vi "Generate Case Description.vi"(8 "error in (no error)":errorcluster, 10 "Test Case Result Out in":T1, 11 "Test Tree In":refnum<class "Test Result Tree.lvclass">) -> (0 "error out":errorcluster, 2 "Test Case Result Out out":T1, 3 "Test Tree Out":refnum<class "Test Result Tree.lvclass">)   [LabVIEW 2020, in "Test Result Tree.lvclass"]
uses:
  Framework/Helper Classes/Test Result Tree/Test Result Tree.lvclass
  Framework/Result Types/Case Result/Test Case Result.ctl
  Framework/Result Types/Method Result/Method Result.ctl
  Result/Status.ctl
  Framework/Result Types/Assertion Result/Assertion Result.ctl
  Framework/Result Types/Assertion Result/Public/TypeDefs/Assertion Type.ctl
  C:/Git/astemes-lunit/source/Framework/Helper Classes/Test Tree/Test Tree.lvclass
  Test Tree.lvclass/Test Tree.ctl
  Framework/Result Types/Case Result/Private/Count by Status.vi
  Framework/Result Types/Case Result/Test Case Result.lvlib
  Test Tree.lvclass
  Framework/Result Types/Assertion Result/Assertion Result.lvlib
  Framework/Result Types/Method Result/Method Result.lvlib
  Result/Result.lvlib
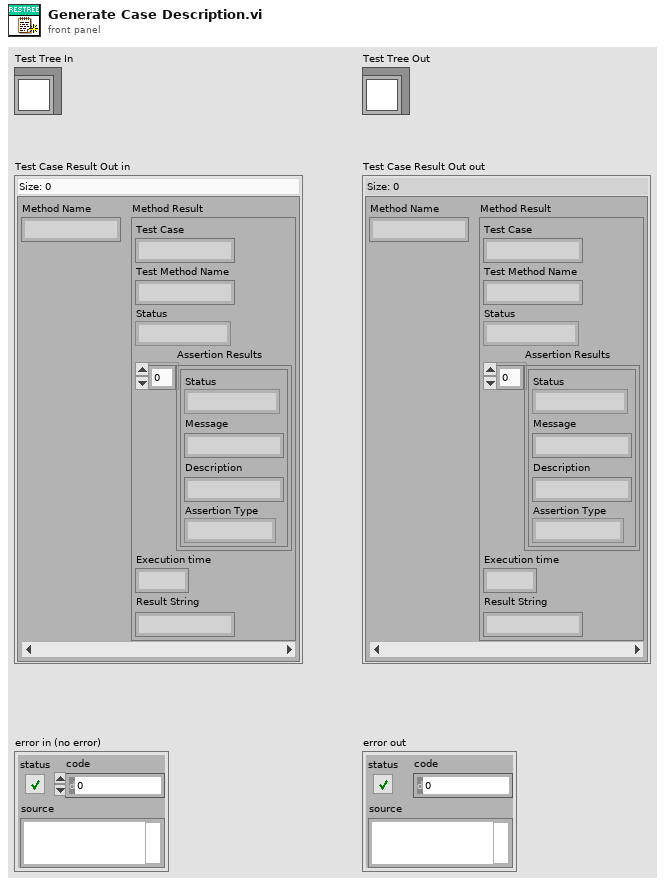
[diagram p1: front panel]
types:
  T1 = typedef "Test Case Result.lvlib/Test Case Result.ctl" = map{string, T2}
  T2 = typedef "Method Result.lvlib/Method Result.ctl" = cluster{"Test Case":string, "Test Method Name":string, "Status":T3, "Assertion Results":T4[], "Execution time":dbl, "Result String":string}
  T3 = typedef "Result.lvlib/Status.ctl" = enum16{"Passed", "Failed", "Error", "Skipped", "Setup Error", "Broken", "Teardown Error"}
  T4 = typedef "Assertion Result.lvlib/Assertion Result.ctl" = cluster{"Status":T3, "Message":string, "Description":string, "Assertion Type":T5}
  T5 = typedef "Result.lvlib/Assertion Type.ctl" = enum16{"None", "Pass", "Fail", "Skip", "Pass if Equal", "Fail if Equal", "Pass if Error", "Fail if Error", "Pass if", "Fail if"}
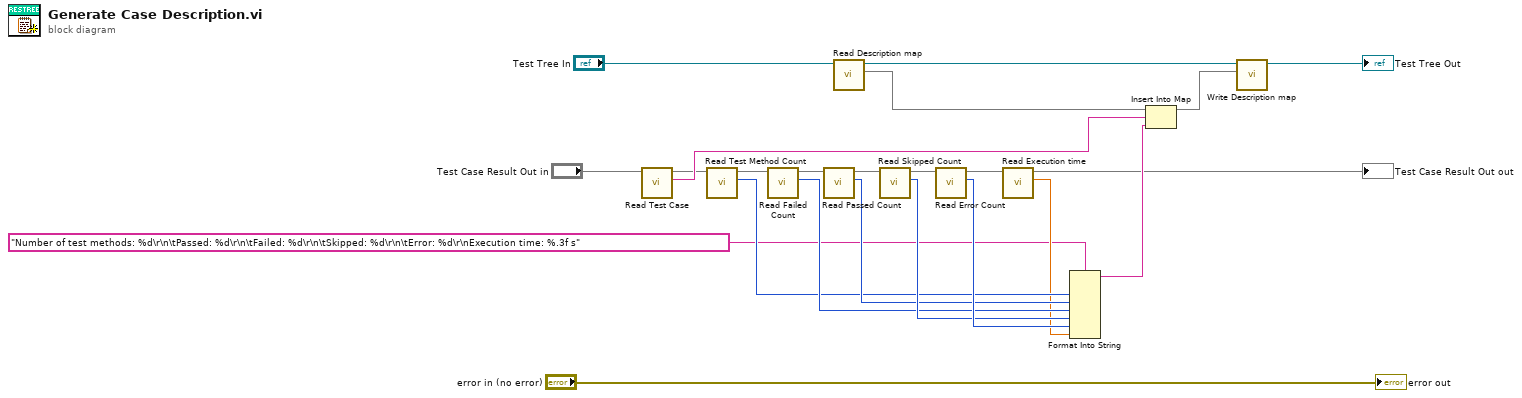
[diagram p0: block diagram]
diagram:
  n1 = call "Read Test Case.vi"("Test Case Result In"="Test Case Result Out in") -> ("Test Case"=w23:string, "Test Case Result Out"=w13:T1)  [unwired: 9 in]
  n2 = call "Read Test Method Count.vi"("Test Case Result In"=w13) -> ("Numeric"=w11:i32, "Test Case Result Out"=w12:T1)  [unwired: 9 in]
  n3 = call "Read Failed Count.vi"("Test Case Result In"=w12) -> ("Fail count"=w18:i32, "Test Case Result Out"=w14:T1)  [unwired: 9 in]
  n4 = call "Read Passed Count.vi"("Test Case Result In"=w14) -> ("Pass count"=w17:i32, "Test Case Result Out"=w15:T1)  [unwired: 9 in]
  n5 = call "Read Description map.vi"("Test Tree in"="Test Tree In") -> ("Description map"=w2:map{string, string}, "Test Tree out"=w5:refnum<class "Test Result Tree.lvclass">)  [unwired: 8 in, 1 out]
  n6 = call "Read Skipped Count.vi"("Test Case Result In"=w15) -> ("Skipped count"=w19:i32, "Test Case Result Out"=w16:T1)  [unwired: 9 in]
  n7 = call "Read Error Count.vi"("Test Case Result In"=w16) -> ("Error count"=w20:i32, "Test Case Result Out"=w10:T1)  [unwired: 9 in]
  n8 = call "Read Execution time.vi"("Test Case Result In"=w10) -> ("Execution time"=w8:dbl, "Test Case Result Out"=→"Test Case Result Out out":T1)  [unwired: 9 in]
  n9 = Format Into String(format string="Number of test methods: %d\r\n\tPassed: %d\r\n\tFailed: %d\r\n\tSkipped: %d\r\n\tError: %d\r\nExecution time: %.3f s", w11, w17, w18, w19, w20, w8) -> (resulting string=w21:string)  [unwired: 2 in, 1 out]
  n10 = Insert Into Map(map in=w2, key=w23, value=w21) -> (map out=w3:map{string, string})  [unwired: 2 out]
  n11 = call "Write Description map.vi"("Description map"=w3, "Test Tree in"=w5) -> ("Test Tree out"=→"Test Tree Out":refnum<class "Test Result Tree.lvclass">)  [unwired: 8 in, 1 out]
  "error out" <- "error in (no error)"
